vi "ACT_Loop.vi"() -> ()   [LabVIEW 2023, in "Template FX_ACT.lvlib"]
uses:
  Template FX_ACT.lvlib
  RoboRIO Utilities/Global_STOP.vi
  ENUM_ACT_Action.ctl
  ENUM_ACT_State.ctl
  Global_CMD_ACT_Data In.vi
  Global_ACT_Data Out.vi
  Cluster_CMD_ACT_Data.ctl
  <vilib>/Rock Robotics/WPI/MotorControl/WPI_MotorControlType.ctl
  <vilib>/Rock Robotics/SystemInterfaces/DIO/FPGA_DIOPWMChannel.ctl
  <vilib>/Rock Robotics/WPI/PWM/WPI_PWMDeadband.ctl
  <vilib>/Rock Robotics/SystemInterfaces/DIO/FPGA_DIOChannel.ctl
  <vilib>/Rock Robotics/WPI/MotorControl/WPI_MotorControlDeviceRef.ctl
  Shared Code/TypeDefs/Cluser_CAN Data.ctl
  <vilib>/Rock Robotics/WPI/ThirdParty/Phoenix-LabVIEW/Motor Controller/Controls/CTRE_Phoenix_MotorControl_NeutralMode.ctl
  Shared Code/TypeDefs/Cluster_FWD  REV Values.ctl
  Shared Code/TypeDefs/Cluster_Config SRX Motor Output.ctl
  Shared Code/TypeDefs/Cluster_PID Gains.ctl
  Shared Code/TypeDefs/Cluster_SRX SLOT PID Config.ctl
  Shared Code/TypeDefs/Cluster_FX Motion Magic Parameters.ctl
  <vilib>/Rock Robotics/WPI/ThirdParty/Phoenix-LabVIEW/Motor Controller/Controls/CTRE_Phoenix_MotorControl_LimitSwitchNormal.ctl
  Shared Code/TypeDefs/Cluser_Hard Limits.ctl
  Shared Code/TypeDefs/Cluser_Enable-Value I32.ctl
  Shared Code/TypeDefs/Cluser_Config_Soft Limits.ctl
  Shared Code/TypeDefs/Cluser_FX Config_Limit Travel.ctl
  Cluster_Config HW Values.ctl
  b5508d6c-c1cc-4273-80c5-2077d34e1483.vi
  5f725c2a-0ce1-4524-8967-e83b15fdce90.vi
  <vilib>/Rock Robotics/WPI/ThirdParty/Phoenix-LabVIEW/Motor Controller/Controls/CTRE_Phoenix_MotorControl_ControlMode.ctl
  Shared Code/TypeDefs/Cluster_FX CloseLoop Values.ctl
  Shared Code/TypeDefs/Cluster_FX Limit Switchs.ctl
  Shared Code/TypeDefs/Cluster_FX Current Values.ctl
  Cluster_HW Output Values.ctl
  ENUM_CMD_Mode Select.ctl
  Shared Code/TypeDefs/Cluster_FX Sensor Values.ctl
  4f1f8321-3dc8-4b28-8619-20673fc77ec2.vi
  Cluster_SW Output Data.ctl
  Cluster_Config SW Values.ctl
  36677ea0-a1a5-47a3-bc56-4475cb7c281e.vi
  573e44c0-11f4-4bd9-ad56-904ec25dba75.vi
  e7494af9-f670-4352-9dfa-ae6ce50709ea.vi
  6201c2b1-dcd8-4430-86f1-9b4ee56c7753.vi
  Shared Code/TypeDefs/Cluser_FX Config_Current Limits.ctl
  Shared Code/TypeDefs/Cluster_FX_HW All Sensor Values.ctl
  Shared Code/TypeDefs/Cluster_FX Output Set Values.ctl
  Shared Code/TypeDefs/Cluster_High-Low.ctl
panel:
  in  "CMD Override":enum32{"None", "Mode 2", "Mode 1", "STOP"}(tab)
  in  "Mode 2 Data":dbl(slide) scale=-0.2..0.2
  in  "Mode 1 Data":i32
  in  "GO":bool
  out "Current Time":timestamp
  in  "SW Config":T1={"Ver"=0, "Config 1"=0.2}
  out "SW Output":T2
  out "Sensor Read time":dbl format="%.3g"
  out "HW Sensors":T3 {"Set"."Mode" items=["PercentOutput"=0, "Position"=1, "Velocity"=2, "Current"=3, "Follower"=5, "MotionProfile"=6, "MotionMagic"=7, "MotionProfileArc"=10, "Disabled"=15]}
  in  "Read Saved Config":bool
  in  "Update Config":bool
  in  "HW Config":T11 {"TravelLimits"."Soft"."REV"."Counts" format="%#.0f"; "TravelLimits"."Soft"."FWD"."Counts" format="%#.0f"; "Output"."Min"."REV" format="%.2f"; "Output"."Min"."FWD" format="%.2f"; "Output"."Max"."REV" format="%.2f"; "Output"."Max"."FWD" format="%.2f"; "CL"."Max I Accu"."Low" format="%#.8f"; "CL"."Max I Accu"."High" format="%#.8f"; "CL"."Gains"."F" format="%#.8f"; "CL"."Gains"."D" format="%#.8f"; "CL"."Gains"."I" format="%#.8f"; "CL"."Gains"."P" format="%#.8f"; "CL"."Error Allowed"."Low" format="%#.8f"; "CL"."Error Allowed"."High" format="%#.8f"; "CL"."I Zone"."Low" format="%#.8f"; "CL"."I Zone"."High" format="%#.8f"; "CL"."Max Out"."REV" format="%.2f"; "CL"."Max Out"."FWD" format="%.2f"}
  out "CMD":T26
  out "Cycle Time (S)":dbl format="%.3g"
  # "STOP"
  # "Tune Output\nto 1023 Max"
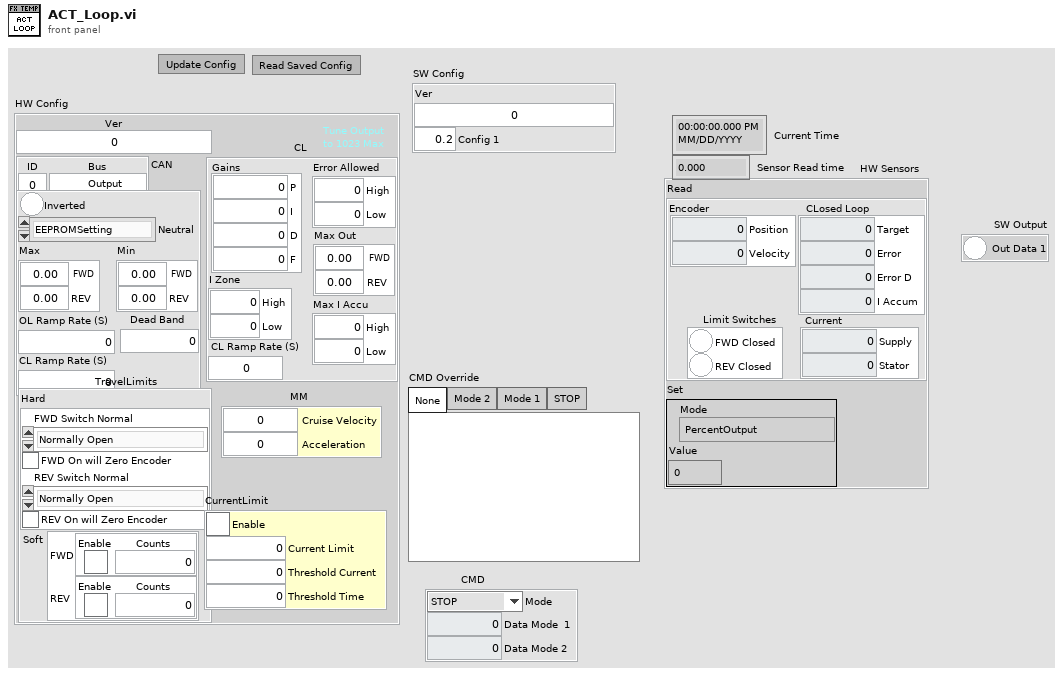
[diagram p1: front panel]
types:
  T1 = typedef "Template FX_ACT.lvlib/Cluster_Config SW Values.ctl" = cluster{"Ver":u64, "Config 1":dbl}
  T2 = typedef "Template FX_ACT.lvlib/Cluster_SW Output Data.ctl" = cluster{"Out Data 1":bool}
  T3 = typedef "Template FX_ACT.lvlib/Cluster_HW Output Values.ctl" = cluster{"Read":T4, "Set":T9}
  T4 = typedef "Cluster_FX_HW All Sensor Values.ctl" = cluster{"Encoder":T5, "CLosed Loop":T6, "Limit Switches":T7, "Current":T8}
  T5 = typedef "Cluster_FX Sensor Values.ctl" = cluster{"Position":i32, "Velocity":i32}
  T6 = typedef "Cluster_FX CloseLoop Values.ctl" = cluster{"Target":dbl, "Error":i32, "Error D":dbl, "I Accum":dbl}
  T7 = typedef "Cluster_FX Limit Switchs.ctl" = cluster{"FWD Closed":bool, "REV Closed":bool}
  T8 = typedef "Cluster_FX Current Values.ctl" = cluster{"Supply":dbl, "Stator":dbl}
  T9 = typedef "Cluster_FX Output Set Values.ctl" = cluster{"Mode":T10, "Value":dbl}
  T10 = typedef "CTRE_Phoenix_MotorControl_ControlMode.ctl" = u16
  T11 = typedef "Template FX_ACT.lvlib/Cluster_Config HW Values.ctl" = cluster{"Ver":u64, "CAN":T12, "Output":T13, "CL":T16, "MM":T19, "TravelLimits":T20, "CurrentLimit":T25}
  T12 = typedef "Cluser_CAN Data.ctl" = cluster{"ID":u8, "Bus":string}
  T13 = typedef "Cluster_Config SRX Motor Output.ctl" = cluster{"Inverted":bool, "Neutral":T14, "Max":T15, "Min":T15, "OL Ramp Rate (S)":dbl, "Dead Band":dbl, "CL Ramp Rate (S)":dbl}
  T14 = typedef "CTRE_Phoenix_MotorControl_NeutralMode.ctl" = enum8{"EEPROMSetting", "Override to Coast", "Override to Brake"}
  T15 = typedef "Cluster_FWD  REV Values.ctl" = cluster{"FWD":dbl, "REV":dbl}
  T16 = typedef "Cluster_PID Config.ctl" = cluster{"Gains":T17, "Error Allowed":T18, "I Zone":T18, "Max Out":T15, "Max I Accu":T18, "CL Ramp Rate (S)":dbl}
  T17 = typedef "Cluster_PID Gains.ctl" = cluster{"P":dbl, "I":dbl, "D":dbl, "F":dbl}
  T18 = typedef "Cluster_High-Low.ctl" = cluster{"High":dbl, "Low":dbl}
  T19 = typedef "Cluster_FX Motion Magic Parameters.ctl" = cluster{"Cruise Velocity":i32, "Acceleration":i32}
  T20 = typedef "Cluser_FX Config_Limit Travel.ctl" = cluster{"Hard":T21, "Soft":T23}
  T21 = typedef "Cluser_Hard Limits.ctl" = cluster{"FWD Switch Normal":T22, "FWD On will Zero Encoder ":bool, "REV Switch Normal":T22, "REV On will Zero Encoder ":bool}
  T22 = typedef "CTRE_Phoenix_MotorControl_LimitSwitchNormal.ctl" = enum16{"Normally Open", "Normally Closed", "Disabled"}
  T23 = typedef "Cluser_Config_Soft Limits.ctl" = cluster{"FWD":T24, "REV":T24}
  T24 = typedef "Cluser_Enable-Value I32.ctl" = cluster{"Enable":bool, "Counts":i32}
  T25 = typedef "Cluser_FX Config_Current Limits.ctl" = cluster{"Enable":bool, "Current Limit":dbl, "Threshold Current":dbl, "Threshold Time":dbl}
  T26 = typedef "Template FX_ACT.lvlib/Cluster_CMD_ACT_Data.ctl" = cluster{"Mode":T27, "Data Mode  1":dbl, "Data Mode 2":dbl}
  T27 = typedef "Template FX_ACT.lvlib/ENUM_CMD_Mode Select.ctl" = enum16{"STOP", "Mode 1", "Mode 2"}
  T28 = typedef "Template FX_ACT.lvlib/Cluster_Config HW Values.ctl" = cluster{"Ver":u64, "CAN":T12, "Output":T29, "CL":T30, "MM":T19, "TravelLimits":T20, "CurrentLimit":T25}
  T29 = typedef "Cluster_Config SRX Motor Output.ctl" = cluster{"Neutral":T14, "Max":T15, "Min":T15, "OL Ramp Rate (S)":dbl, "Dead Band":dbl, "CL Ramp Rate (S)":dbl}
  T30 = typedef "Cluster_SRX SLOT PID Config.ctl" = cluster{"Gains":T17, "Error Allowed":dbl, "I Zone":dbl, "Peak Out 0-1":dbl, "Max I Accu":dbl}
  T31 = typedef "Template FX_ACT.lvlib/ENUM_ACT_State.ctl" = enum16{"Startup", "Configuring", "Stopping", "Moving Mode 1", "Moving Mode 2", "Shutdown"}
  T32 = typedef "WPI_MotorControlDeviceRef.ctl" = cluster{"DeviceStatus":errorcluster, "Type":T33, "PWM":cluster{"PWM Channel":T34, "DeadBand":T35}, "CAN":cluster{"Device Number":u8, "SetOutput VI Ref":variant, "GetOutput VI Ref":variant, "Enable VI Ref":variant, "Disable VI Ref":variant, "Data":variant}, "Invert":bool, "DIO PWM":cluster{"PWM \"Enable\" Channel":T34, "DIOChannel":T36, "PWM Rate":dbl}}
  T33 = typedef "WPI_MotorControlType.ctl" = enum16{"PWM", "CAN", "DIO PWM"}
  T34 = typedef "FPGA_DIOPWMChannel.ctl" = enum8{"PWM 0", "PWM 1", "PWM 2", "PWM 3", "PWM 4", "PWM 5", "PWM 6", "PWM 7", "PWM 8", "PWM 9", "PWM MXP 0", "PWM MXP 1", "PWM MXP 2", "PWM MXP 3", "PWM MXP 4", "PWM MXP 5", "PWM MXP 6", "PWM MXP 7", "PWM MXP 8", "PWM MXP 9", "Invalid"}
  T35 = typedef "WPI_PWMDeadband.ctl" = cluster{"Name":string, "maxPositivePwm":i32, "minPositivePwm":i32, "centerPwm":i32, "maxNegativePwm":i32, "minNegativePwm":i32, "angularRange":u16}
  T36 = typedef "FPGA_DIOChannel.ctl" = enum8{"DIO 0", "DIO 1", "DIO 2", "DIO 3", "DIO 4", "DIO 5", "DIO 6", "DIO 7", "DIO 8", "DIO 9", "DIO MXP 0", "DIO MXP 1", "DIO MXP 2", "DIO MXP 3", "DIO MXP 4", "DIO MXP 5", "DIO MXP 6", "DIO MXP 7", "DIO MXP 8", "DIO MXP 9", "DIO MXP 10", "DIO MXP 11", "DIO MXP 12", "DIO MXP 13", "DIO MXP 14", "DIO MXP 15", "SPI Port CS1", "SPI Port CS2", "SPI Port CS3", "SPI Port MISO", "SPI Port MOSI", "Invalid"}
  T37 = cluster{"Team Files Folder":path, "FX Ref":T32, "State":T31, "Previous State":T31, "Current Time":timestamp, "Previous Time":timestamp, "Start Time":timestamp, "Target Time (ms)":u32, "Cycle Time(S)":dbl, "Update Display":bool, "ACT Input":T26, "HW Config":T28, "SW Config":T1, "Max # Of Config Tries":i32, "HW Out":T3, "SW Out":T2, "CAN Timeout":u32, "FX Mode":T10, "FX Set Value":dbl}
  T38 = typedef "Template FX_ACT.lvlib/ENUM_ACT_Action.ctl" = enum16{"No Action", "Reset Time", "Reset All", "Config HW File Read", "Config HW File Save", "Config SW File Read", "Config SW File Save", "Config From FP", "Config HW Get", "Config HW Set", "Open HW Only", "Control FX Stop", "Control FX Mode 1", "Control FX Mode 2"}
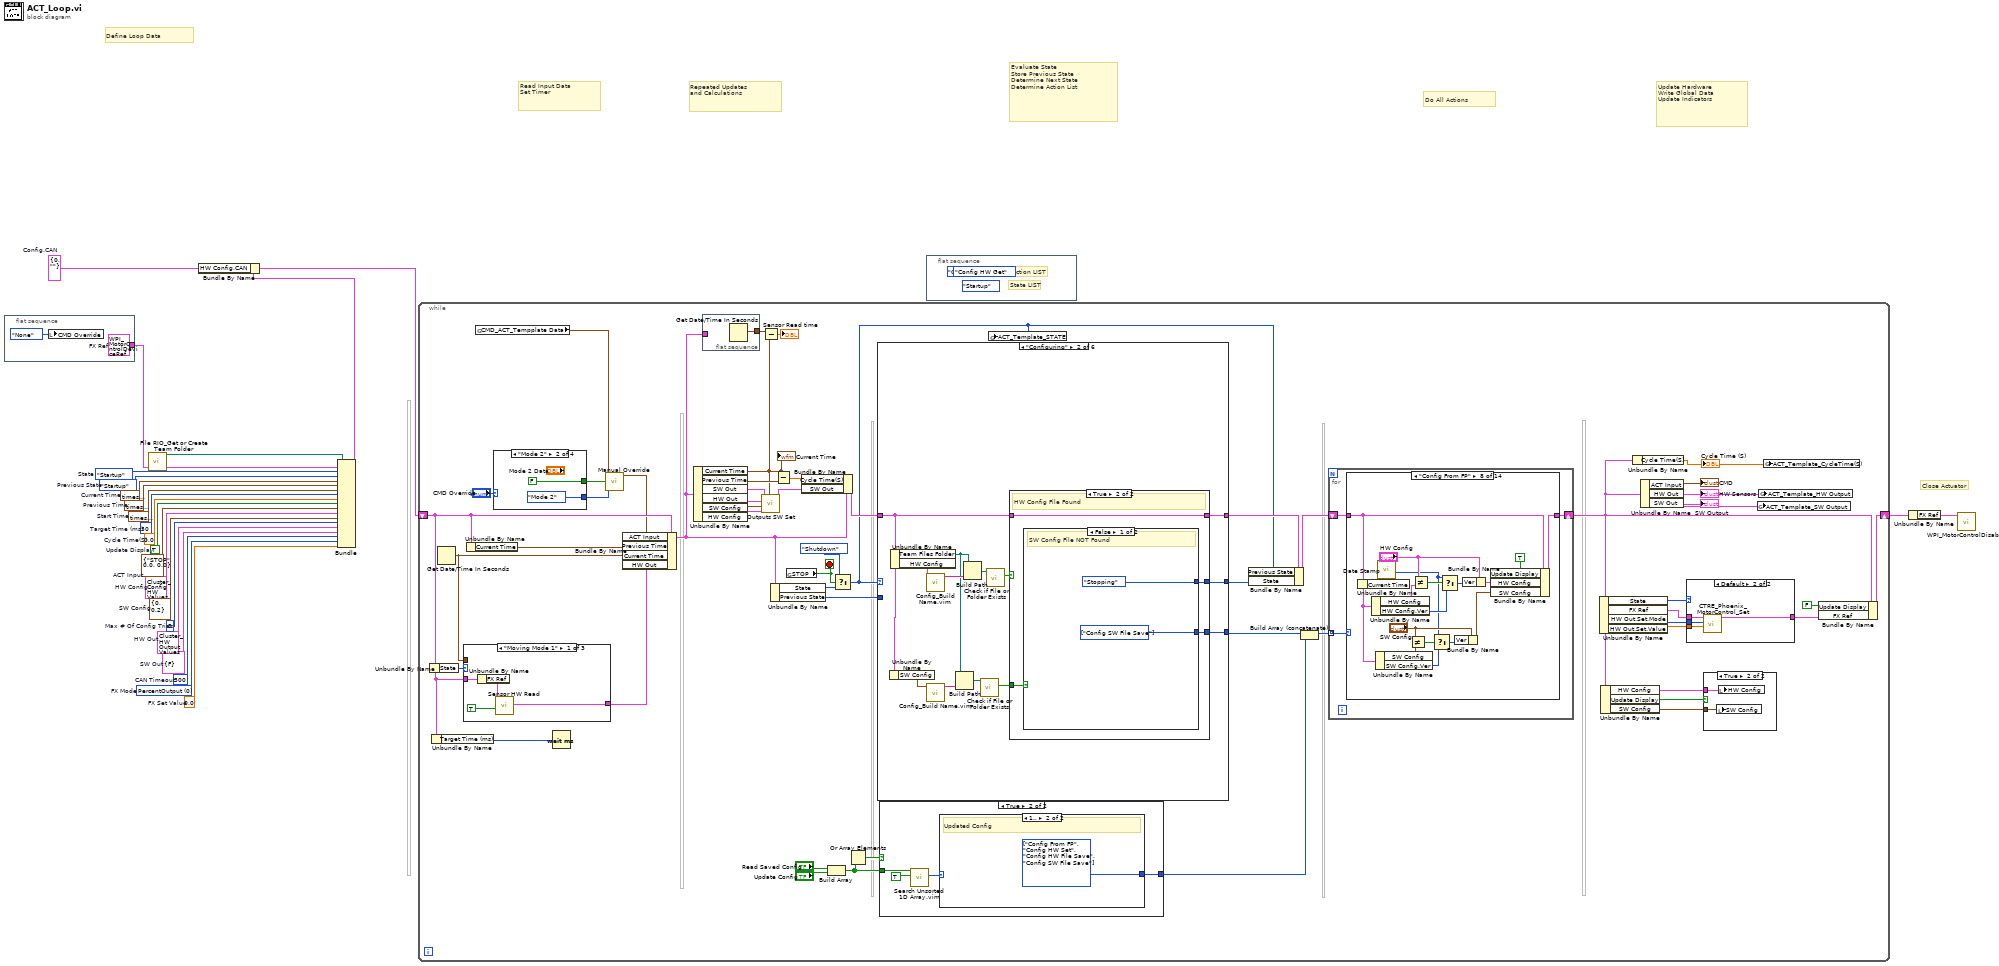
[diagram p0: block diagram]
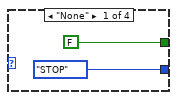
[diagram p2: hidden frame]
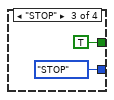
[diagram p3: hidden frame]
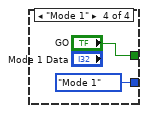
[diagram p4: hidden frame]
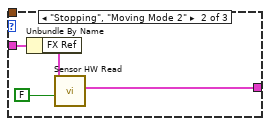
[diagram p5: hidden frame]
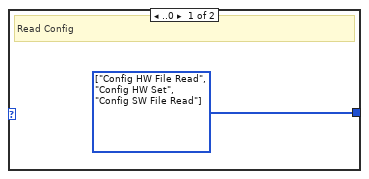
[diagram p8: hidden frame]
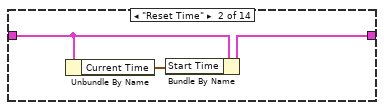
[diagram p10: hidden frame]
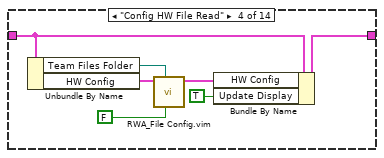
[diagram p12: hidden frame]
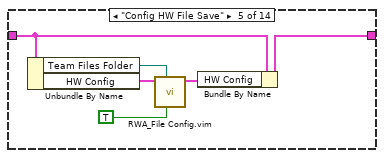
[diagram p13: hidden frame]
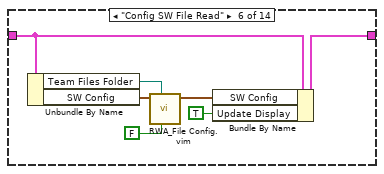
[diagram p14: hidden frame]
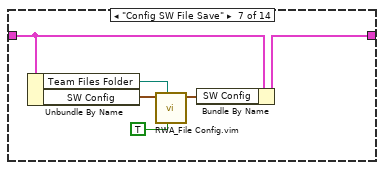
[diagram p15: hidden frame]
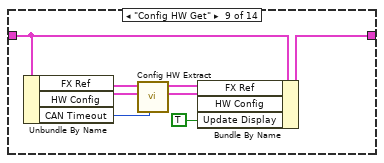
[diagram p16: hidden frame]
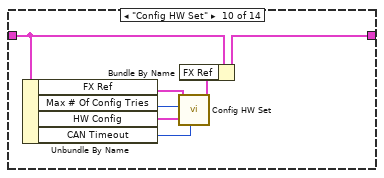
[diagram p17: hidden frame]
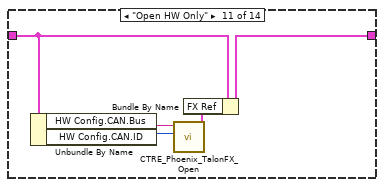
[diagram p18: hidden frame]
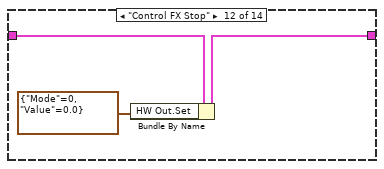
[diagram p19: hidden frame]
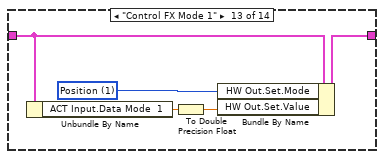
[diagram p20: hidden frame]
diagram:
  w10 = T28 {"Ver"=0, "CAN"={"ID"=0, "Bus"=""}, "Output"={"Neutral"=enum."EEPROMSetting", "Max"={"FWD"=0.0, "REV"=0.0}, "Min"={"FWD"=0.0, "REV"=0.0}, "OL Ramp Rate (S)"=0.0, "Dead Band"=0.0, "CL Ramp Rate (S)"=0.0}, "CL"={"Gains"={"P"=0.0, "I"=0.0, "D"=0.0, "F"=0.0}, "Error Allowed"=0.0, "I Zone"=0.0, "Peak Out 0-1"=0.0, "Max I Accu"=0.0}, "MM"={"Cruise Velocity"=0, "Acceleration"=0}, "TravelLimits"={"Hard"={"FWD Switch Normal"=enum."Normally Open", "FWD On will Zero Encoder "=FALSE, "REV Switch Normal"=enum."Normally Open", "REV On will Zero Encoder "=FALSE}, "Soft"={"FWD"={"Enable"=FALSE, "Counts"=0}, "REV"={"Enable"=FALSE, "Counts"=0}}}, "CurrentLimit"={"Enable"=FALSE, "Current Limit"=0.0, "Threshold Current"=0.0, "Threshold Time"=0.0}}  # HW Config
  w7 = T2 {"Out Data 1"=FALSE}  # SW Out
  w9 = T1 {"Ver"=0, "Config 1"=0.2}  # SW Config
  w8 = T3 {"Read"={"Encoder"={"Position"=0, "Velocity"=0}, "CLosed Loop"={"Target"=0.0, "Error"=0, "Error D"=0.0, "I Accum"=0.0}, "Limit Switches"={"FWD Closed"=FALSE, "REV Closed"=FALSE}, "Current"={"Supply"=0.0, "Stator"=0.0}}, "Set"={"Mode"=0, "Value"=0.0}}  # HW Out
  w3 = 0.0  # FX Set Value
  w4 = T10 0 items=["PercentOutput"=0, "Position"=1, "Velocity"=2, "Current"=3, "Follower"=5, "MotionProfile"=6, "MotionMagic"=7, "MotionProfileArc"=10, "Disabled"=15]  # FX Mode
  w2 = u32 300  # CAN Timeout
  w1 = 3  # Max # Of Config Tries
  w12 = TRUE  # Update Display
  w13 = T12 {"ID"=0, "Bus"=""}  # Config.CAN
  w18 = 0.0  # Cycle Time(S)
  w19 = ENUM_ACT_State."Startup"  # Previous State
  w20 = timestamp(0 s since 1904-01-01)  # Previous Time
  w21 = u32 50  # Target Time (ms)
  w6 = T26 {"Mode"=enum."STOP", "Data Mode  1"=0.0, "Data Mode 2"=0.0}  # ACT Input
  w22 = timestamp(0 s since 1904-01-01)  # Start Time
  w23 = timestamp(0 s since 1904-01-01)  # Current Time
  w24 = ENUM_ACT_State."Startup"  # State
  # "Close Actuator"
  # "Define Loop Data"
  # "Repeated Updates\nand Calculations"
  # "Read Input Data\nSet Timer"
  # "Evaluate State\nStore Previous State\nDetermine Next State\nDetermine Action List"
  # "Do All Actions"
  # "Update Hardware\nWrite Global Data\nUpdate Indicators"
  n1 = flat-sequence {
    tunnel: [w26] -> w14
    frame #0 {
      w26 = T32 {"DeviceStatus"={"status"=FALSE, "code"=0, "source"=""}, "Type"=enum."PWM", "PWM"={"PWM Channel"=enum."PWM 1", "DeadBand"={"Name"="", "maxPositivePwm"=0, "minPositivePwm"=0, "centerPwm"=0, "maxNegativePwm"=0, "minNegativePwm"=0, "angularRange"=0}}, "CAN"={"Device Number"=0, "SetOutput VI Ref"=variant(enum8{"Percent VBus", "Current", "Speed", "Position", "Voltage"} enum."Percent VBus"), "GetOutput VI Ref"=variant(refnum<k1> refnum), "Enable VI Ref"=variant(dbl 12.0), "Disable VI Ref"=variant(enum8{"Percent VBus", "Speed", "Position", "Slave", "Unchanged / Invalid", "Voltage Compensation", "Current", "Motion Profile"} enum."Percent VBus"), "Data"=variant}, "Invert"=FALSE, "DIO PWM"={"PWM \"Enable\" Channel"=enum."Invalid", "DIOChannel"=enum."Invalid", "PWM Rate"=0.0}}  # FX Ref
      n2 = local write "CMD Override"(enum32{"None", "Mode 2", "Mode 1", "STOP"}."None" ("CMD Override")) -> ()
    }
  }
  n3 = call "File RIO_Get or Create Team Folder.vi"() -> ("Team Files Folder"=w5:path)  [unwired: 10 in, 1 out]
  n4 = Bundle("Team Files Folder"=w5, "FX Ref"=w14, "State"=w24, "Previous State"=w19, "Current Time"=w23, "Previous Time"=w20, "Start Time"=w22, "Target Time (ms)"=w21, "Cycle Time(S)"=w18, "Update Display"=w12, "ACT Input"=w6, "HW Config"=w10, "SW Config"=w9, "Max # Of Config Tries"=w1, "HW Out"=w8, "SW Out"=w7, "CAN Timeout"=w2, "FX Mode"=w4, "FX Set Value"=w3) -> (w16:T37)  [unwired: 1 in]
  n5 = Bundle By Name(cluster=w16, "HW Config.CAN"=w13) -> (w15:T37)
  n6 = while {
    shift-right: [w63] -> w17
    shift-left: w15 -> [w33]
    stop <- w76 stop-if-true
    n7 = Unbundle By Name(w33) -> ("State"=w53:T31)
    n8 = Unbundle By Name(w33) -> ("Target Time (ms)"=w73:u32)
    n9 = Get Date/Time In Seconds() -> (seconds since 1Jan1904=w49:timestamp)
    n10 = case shown="\"Moving Mode 1\"" w53 {
      tunnel: w33 -> [w92 w96 _]
      tunnel: w49 -> [_ _ _]
      tunnel: [w89 w93 _] -> w34
      frame "Moving Mode 1" {
        n11 = Unbundle By Name(w92) -> ("FX Ref"=w91:T32)
        n12 = call "Sensor HW Read.vi"("Read Closed Loop"=TRUE, "Ref"=w91) -> ("Sensor Values Out"=w89:T3)  [unwired: 7 in, 2 out]
      }
      frame "Stopping", "Moving Mode 2" {
        n13 = Unbundle By Name(w96) -> ("FX Ref"=w95:T32)
        n14 = call "Sensor HW Read.vi"("Read Closed Loop"=FALSE, "Ref"=w95) -> ("Sensor Values Out"=w93:T3)  [unwired: 7 in, 2 out]
      }
      frame "Startup", "Configuring", "Shutdown" {
      }
    }
    n15 = Unbundle By Name(w33) -> ("Current Time"=w72:timestamp)
    n16 = global read "Global_CMD_ACT_Data In.vi" "CMD_ACT_Tempplate Data"() -> (w31:T26)
    n17 = case shown="\"Mode 2\"" "CMD Override" {
      tunnel: [FALSE ("Enable") FALSE ("Enable") TRUE ("Positon GO") "GO"] -> w29
      tunnel: [ENUM_CMD_Mode_Select."STOP" ("Override") ENUM_CMD_Mode_Select."Mode 2" ("Override") ENUM_CMD_Mode_Select."STOP" ("Override") ENUM_CMD_Mode_Select."Mode 1" ("Override")] -> w28
      frame "None" {
      }
      frame "Mode 2" {
      }
      frame "STOP" {
      }
      frame "Mode 1" {
      }
    }
    n18 = Wait (ms)(milliseconds to wait=w73) -> ()  [unwired: 1 out]
    n19 = call "Manual Override.vi"("Override"=w28, "Enable"=w29, "Auto CMD"=w31) -> ("OverRide Command Out"=w32:T26)  [unwired: 8 in]
    n20 = Bundle By Name(cluster=w33, "ACT Input"=w32, "Previous Time"=w72, "Current Time"=w49, "HW Out"=w34) -> (w35:T37)
    n21 = Unbundle By Name(w35) -> ("Current Time"=w39:timestamp, "Previous Time"=w70:timestamp, "SW Out"=w42:T2, "HW Out"=w40:T3, "SW Config"=w38:T1, "HW Config"=w37:T28)
    "Current Time" <- w39
    n22 = flat-sequence {
      tunnel: [w88] -> w51
      tunnel: w35 -> [_]
      frame #0 {
        n23 = Get Date/Time In Seconds() -> (seconds since 1Jan1904=w88:timestamp)
      }
    }
    n24 = call "Outputs SW Set.vi"("Current Time"=w39, "HW Config"=w37, "SW Config"=w38, "Sensor Values"=w40, "SW Output"=w42) -> ("SW Output Out"=w41:T2)  [unwired: 6 in]
    n25 = Subtract(x=w51, y=w39) -> (x-y=→"Sensor Read time":dbl)
    n26 = Unbundle By Name(w35) -> ("State"=w74:T31, "Previous State"=w71:T31)
    n27 = Subtract(x=w39, y=w70) -> (x-y=w68:dbl)
    n28 = global read "Global_STOP.vi" "STOP"() -> (w76:bool)
    n29 = Bundle By Name(cluster=w35, "Cycle Time(S)"=w68, "SW Out"=w41) -> (w69:T37)
    n30 = Build Array("Read Saved Config", "Update Config") -> (w45:bool[])
    n31 = Select(t=ENUM_ACT_State."Shutdown" ("State"), s=w76, f=w74) -> (s? t:f=w27:T31)
    n32 = Or Array Elements(Boolean array=w45) -> (logical OR=w46:bool)
    n33 = case shown="\"Configuring\"" w27 {
      selector: w27 -> [_ _ _ w230 w246 _]
      tunnel: w69 -> [w188 w194 w217 w231 w247 w262]
      tunnel: [w188 w197 w216 w232 w248 w262] -> w78
      tunnel: [ENUM_ACT_State."Configuring" ("State") w196 w215 w234 w250 ENUM_ACT_State."Shutdown" ("State")] -> w77
      tunnel: [w187 w195 w213 w229 w244 w260] -> w67
      tunnel: w71 -> [_ _ _ _ _ _]
      frame "Startup" {
        w187 = T38[] [enum."Reset Time"] items=["No Action", "Reset Time", "Reset All", "Config HW File Read", "Config HW File Save", "Config SW File Read", "Config SW File Save", "Config From FP", "Config HW Get", "Config HW Set", "Open HW Only", "Control FX Stop", "Control FX Mode 1", "Control FX Mode 2"] ("Actions")
      }
      frame "Configuring" {
        n34 = Unbundle By Name(w194) -> ("SW Config"=w192:T1)
        n35 = Unbundle By Name(w194) -> ("Team Files Folder"=w191:path, "HW Config"=w199:T28)
        n36 = call "Config_Build Name.vim"("Config First Name"=w199) -> ("Cfg file"=w201:string)  [unwired: 9 in, 1 out]
        n37 = call "Config_Build Name.vim"("Config First Name"=w192) -> ("Cfg file"=w193:string)  [unwired: 9 in, 1 out]
        n38 = Build Path(base path=w191, name or relative path=w193) -> (appended path=w190:path)
        n39 = Build Path(base path=w191, name or relative path=w201) -> (appended path=w200:path)
        n40 = call <vilib>:"Check if File or Folder Exists.vi"("path"=w190) -> ("file or folder exists?"=w189:bool)  [unwired: 8 in, 2 out]
        n41 = call <vilib>:"Check if File or Folder Exists.vi"("path"=w200) -> ("file or folder exists?"=w198:bool)  [unwired: 8 in, 2 out]
        n42 = case shown="True" w198 {
          tunnel: w194 -> [w204 w208]
          tunnel: [w204 w208] -> w197
          tunnel: [ENUM_ACT_State."Configuring" ("State") w207] -> w196
          tunnel: [w202 w206] -> w195
          tunnel: w189 -> [_ w205]
          frame False {
            w202 = T38[] [enum."Open HW Only", enum."Config HW Get", enum."Config HW File Save"] items=["No Action", "Reset Time", "Reset All", "Config HW File Read", "Config HW File Save", "Config SW File Read", "Config SW File Save", "Config From FP", "Config HW Get", "Config HW Set", "Open HW Only", "Control FX Stop", "Control FX Mode 1", "Control FX Mode 2"] ("Actions")
            # "HW Config File Not Found"
          }
          frame True {
            # "HW Config File Found"
            n43 = case shown="False" w205 {
              tunnel: [ENUM_ACT_State."Stopping" ("State") ENUM_ACT_State."Stopping" ("State")] -> w207
              tunnel: [w209 w211] -> w206
              frame False {
                w209 = T38[] [enum."Config SW File Save"] items=["No Action", "Reset Time", "Reset All", "Config HW File Read", "Config HW File Save", "Config SW File Read", "Config SW File Save", "Config From FP", "Config HW Get", "Config HW Set", "Open HW Only", "Control FX Stop", "Control FX Mode 1", "Control FX Mode 2"] ("Actions")
                # "SW Config File NOT Found"
              }
              frame True {
                w211 = T38[] [enum."Config HW File Read", enum."Config HW Set", enum."Config SW File Read", enum."Reset All", enum."Control FX Stop"] items=["No Action", "Reset Time", "Reset All", "Config HW File Read", "Config HW File Save", "Config SW File Read", "Config SW File Save", "Config From FP", "Config HW Get", "Config HW Set", "Open HW Only", "Control FX Stop", "Control FX Mode 1", "Control FX Mode 2"] ("Actions")
                # "SW Config File Found"
              }
            }
          }
        }
      }
      frame "Stopping" {
        (unwired) TRUE
        w214 = T38[] [enum."Control FX Stop"] items=["No Action", "Reset Time", "Reset All", "Config HW File Read", "Config HW File Save", "Config SW File Read", "Config SW File Save", "Config From FP", "Config HW Get", "Config HW Set", "Open HW Only", "Control FX Stop", "Control FX Mode 1", "Control FX Mode 2"] ("Actions")
        n44 = Unbundle By Name(w217) -> ("ACT Input.Mode"=w218:T27)
        n45 = case shown="\"STOP\"" w218 {
          tunnel: w217 -> [w221 w224 w227]
          tunnel: [w221 w224 w227] -> w216
          tunnel: [ENUM_ACT_State."Stopping" ("State") ENUM_ACT_State."Moving Mode 1" ("State") ENUM_ACT_State."Moving Mode 2" ("State")] -> w215
          tunnel: [w219 w222 w225] -> w213
          tunnel: w214 -> [w219 w222 w225]
          frame "STOP" {
          }
          frame "Mode 1" {
          }
          frame "Mode 2" {
          }
        }
      }
      frame "Moving Mode 1" {
        w228 = T38[] [enum."Control FX Stop"] items=["No Action", "Reset Time", "Reset All", "Config HW File Read", "Config HW File Save", "Config SW File Read", "Config SW File Save", "Config From FP", "Config HW Get", "Config HW Set", "Open HW Only", "Control FX Stop", "Control FX Mode 1", "Control FX Mode 2"] ("Actions")
        n46 = Unbundle By Name(w231) -> ("ACT Input.Mode"=w233:T27)
        n47 = case shown="\"Mode 2\"" w233 {
          tunnel: [ENUM_ACT_State."Stopping" ("State") ENUM_ACT_State."Moving Mode 2" ("State") w242] -> w234
          tunnel: w231 -> [w237 w240 w243]
          tunnel: [w237 w240 w243] -> w232
          tunnel: w230 -> [_ _ w242]
          tunnel: [w235 w238 w241] -> w229
          tunnel: w228 -> [w235 w238 _]
          frame "STOP" {
          }
          frame "Mode 2" {
          }
          frame "Mode 1" {
            w241 = T38[] [enum."Control FX Mode 1"] items=["No Action", "Reset Time", "Reset All", "Config HW File Read", "Config HW File Save", "Config SW File Read", "Config SW File Save", "Config From FP", "Config HW Get", "Config HW Set", "Open HW Only", "Control FX Stop", "Control FX Mode 1", "Control FX Mode 2"] ("Actions")
          }
        }
      }
      frame "Moving Mode 2" {
        w245 = T38[] [enum."Control FX Stop"] items=["No Action", "Reset Time", "Reset All", "Config HW File Read", "Config HW File Save", "Config SW File Read", "Config SW File Save", "Config From FP", "Config HW Get", "Config HW Set", "Open HW Only", "Control FX Stop", "Control FX Mode 1", "Control FX Mode 2"] ("Actions")
        n48 = Unbundle By Name(w247) -> ("ACT Input.Mode"=w249:T27)
        n49 = case shown="\"Mode 2\"" w249 {
          tunnel: [ENUM_ACT_State."Stopping" ("State") w254 ENUM_ACT_State."Moving Mode 1" ("State")] -> w250
          tunnel: w247 -> [w253 w256 w259]
          tunnel: [w253 w256 w259] -> w248
          tunnel: w246 -> [_ w254 _]
          tunnel: [w251 w255 w257] -> w244
          tunnel: w245 -> [w251 _ w257]
          frame "STOP" {
          }
          frame "Mode 2" {
            w255 = T38[] [enum."Control FX Mode 2"] items=["No Action", "Reset Time", "Reset All", "Config HW File Read", "Config HW File Save", "Config SW File Read", "Config SW File Save", "Config From FP", "Config HW Get", "Config HW Set", "Open HW Only", "Control FX Stop", "Control FX Mode 1", "Control FX Mode 2"] ("Actions")
          }
          frame "Mode 1" {
          }
        }
      }
      frame "Shutdown" {
        w260 = T38[] [enum."Reset All"] items=["No Action", "Reset Time", "Reset All", "Config HW File Read", "Config HW File Save", "Config SW File Read", "Config SW File Save", "Config From FP", "Config HW Get", "Config HW Set", "Open HW Only", "Control FX Stop", "Control FX Mode 1", "Control FX Mode 2"] ("Actions")
      }
    }
    n50 = case shown="True" w46 {
      tunnel: w45 -> [_ w99]
      tunnel: [_ w97] -> w44
      frame False {
      }
      frame True {
        n51 = call "Search Unsorted 1D Array.vim"("element"=TRUE, "unsorted 1D array"=w99) -> ("index of element"=w98:i32)  [unwired: 9 in]
        n52 = case shown="1.." w98 {
          tunnel: [w101 w102] -> w97
          frame ..0 {
            w101 = T38[] [enum."Config HW File Read", enum."Config HW Set", enum."Config SW File Read"] items=["No Action", "Reset Time", "Reset All", "Config HW File Read", "Config HW File Save", "Config SW File Read", "Config SW File Save", "Config From FP", "Config HW Get", "Config HW Set", "Open HW Only", "Control FX Stop", "Control FX Mode 1", "Control FX Mode 2"] ("Actions")
            # "Read Config"
          }
          frame 1.. {
            w102 = T38[] [enum."Config From FP", enum."Config HW Set", enum."Config HW File Save", enum."Config SW File Save"] items=["No Action", "Reset Time", "Reset All", "Config HW File Read", "Config HW File Save", "Config SW File Read", "Config SW File Save", "Config From FP", "Config HW Get", "Config HW Set", "Open HW Only", "Control FX Stop", "Control FX Mode 1", "Control FX Mode 2"] ("Actions")
            # "Updated Config"
          }
        }
      }
    }
    n53 = global write "Global_ACT_Data Out.vi" "ACT_Template_STATE"(w27) -> ()
    n54 = Bundle By Name(cluster=w78, "Previous State"=w27, "State"=w77) -> (w79:T37)
    n55 = Build Array (concatenate)(w67, w44) -> (w61:T38[])
    n56 = for {
      tunnel: w61 -> [w105] mode=indexing
      shift-right: [w104] -> w60
      shift-left: w79 -> [w103]
      n57 = case shown="\"Config From FP\"" w105 {
        tunnel: w103 -> [w106 w109 w110 w116 w122 w129 w135 w143 w158 w166 w170 w175 w179 w183]
        tunnel: [w106 w108 w110 w117 w123 w130 w136 w153 w159 w167 w171 w176 w181 w185] -> w104
        frame "No Action" {
        }
        frame "Reset Time" {
          n58 = Unbundle By Name(w109) -> ("Current Time"=w107:timestamp)
          n59 = Bundle By Name(cluster=w109, "Start Time"=w107) -> (w108:T37)
        }
        frame "Reset All" {
        }
        frame "Config HW File Read" {
          n60 = Unbundle By Name(w116) -> ("Team Files Folder"=w113:path, "HW Config"=w115:T28)
          n61 = call "RWA_File Config.vim"("Read(f) Save(t)"=FALSE ("Read(f) Write(t)"), "Target Folder Folder"=w113, "Any Config"=w115) -> ("Any Config Out"=w114:T28)  [unwired: 4 in, 4 out]
          n62 = Bundle By Name(cluster=w116, "HW Config"=w114, "Update Display"=TRUE) -> (w117:T37)
        }
        frame "Config HW File Save" {
          n63 = Unbundle By Name(w122) -> ("Team Files Folder"=w119:path, "HW Config"=w121:T28)
          n64 = call "RWA_File Config.vim"("Read(f) Save(t)"=TRUE ("Read(f) Write(t)"), "Target Folder Folder"=w119, "Any Config"=w121) -> ("Any Config Out"=w120:T28)  [unwired: 4 in, 4 out]
          n65 = Bundle By Name(cluster=w122, "HW Config"=w120) -> (w123:T37)
        }
        frame "Config SW File Read" {
          n66 = Unbundle By Name(w129) -> ("Team Files Folder"=w126:path, "SW Config"=w128:T1)
          n67 = call "RWA_File Config.vim"("Read(f) Save(t)"=FALSE ("Read(f) Write(t)"), "Target Folder Folder"=w126, "Any Config"=w128) -> ("Any Config Out"=w127:T1)  [unwired: 4 in, 4 out]
          n68 = Bundle By Name(cluster=w129, "SW Config"=w127, "Update Display"=TRUE) -> (w130:T37)
        }
        frame "Config SW File Save" {
          n69 = Unbundle By Name(w135) -> ("Team Files Folder"=w132:path, "SW Config"=w134:T1)
          n70 = call "RWA_File Config.vim"("Read(f) Save(t)"=TRUE ("Read(f) Write(t)"), "Target Folder Folder"=w132, "Any Config"=w134) -> ("Any Config Out"=w133:T1)  [unwired: 4 in, 4 out]
          n71 = Bundle By Name(cluster=w135, "SW Config"=w133) -> (w136:T37)
        }
        frame "Config From FP" {
          n72 = Unbundle By Name(w143) -> ("Current Time"=w152:timestamp)
          n73 = Unbundle By Name(w143) -> ("HW Config"=w142:T28, "HW Config.Ver"=w139:u64)
          n74 = Unbundle By Name(w143) -> ("SW Config"=w145:T1, "SW Config.Ver"=w147:u64)
          n75 = call "Date Stamp.vi"("Time"=w152) -> ("U64 Out"=w138:u64)  [unwired: 5 in, 1 out]
          n76 = Not Equal?(x=w145, y="SW Config") -> (x != y?=w148:bool)
          n77 = Not Equal?(x="HW Config", y=w142) -> (x != y?=w140:bool)
          n78 = Select(t=w138, s=w148, f=w147) -> (s? t:f=w146:u64)
          n79 = Select(t=w138, s=w140, f=w139) -> (s? t:f=w137:u64)
          n80 = Bundle By Name(cluster="SW Config", "Ver"=w146) -> (w150:T1)
          n81 = Bundle By Name(cluster="HW Config", "Ver"=w137) -> (w151:T11)
          n82 = Bundle By Name(cluster=w143, "Update Display"=TRUE, "HW Config"=w151, "SW Config"=w150) -> (w153:T37)
        }
        frame "Config HW Get" {
          n83 = Unbundle By Name(w158) -> ("FX Ref"=w161:T32, "HW Config"=w160:T28, "CAN Timeout"=w154:u32)
          n84 = call "Config HW Extract.vi"("Send Cmd Timout(ms)"=w154, "Wrist Config"=w160, "DevRef"=w161) -> ("Wrist Config Data Out"=w156:T11, "DevRef Out"=w157:T32)  [unwired: 6 in, 1 out]
          n85 = Bundle By Name(cluster=w158, "FX Ref"=w157, "HW Config"=w156, "Update Display"=TRUE) -> (w159:T37)
        }
        frame "Config HW Set" {
          n86 = Unbundle By Name(w166) -> ("FX Ref"=w168:T32, "Max # Of Config Tries"=w162:i32, "HW Config"=w164:T28, "CAN Timeout"=w163:u32)
          n87 = call "Config HW Set.vi"("Send Cmd Timout(ms)"=w163, "Wrist Config"=w164, "Max # Of Tries"=w162, "DevRef"=w168) -> ("DevRef Out Out"=w165:T32)  [unwired: 6 in, 1 out]
          n88 = Bundle By Name(cluster=w166, "FX Ref"=w165) -> (w167:T37)
        }
        frame "Open HW Only" {
          n89 = Unbundle By Name(w170) -> ("HW Config.CAN.Bus"=w169:string, "HW Config.CAN.ID"=w173:u8)
          n90 = call <vilib>:"CTRE_Phoenix_TalonFX_Open.vi"("Device Number"=w173, "CAN Bus"=w169) -> ("PhoenixMotorControlDevRef"=w172:T32)  [unwired: 8 in, 1 out]
          n91 = Bundle By Name(cluster=w170, "FX Ref"=w172) -> (w171:T37)
        }
        frame "Control FX Stop" {
          n92 = Bundle By Name(cluster=w175, "HW Out.Set"=T9 {"Mode"=0, "Value"=0.0}) -> (w176:T37)
        }
        frame "Control FX Mode 1" {
          w180 = T10 1 items=["PercentOutput"=0, "Position"=1, "Velocity"=2, "Current"=3, "Follower"=5, "MotionProfile"=6, "MotionMagic"=7, "MotionProfileArc"=10, "Disabled"=15] ("FX Mode")
          n93 = Unbundle By Name(w179) -> ("ACT Input.Data Mode  1"=w177:dbl)
          n94 = To Double Precision Float(number=w177) -> (double precision float=w178:dbl)
          n95 = Bundle By Name(cluster=w179, "HW Out.Set.Mode"=w180, "HW Out.Set.Value"=w178) -> (w181:T37)
        }
        frame "Control FX Mode 2" {
          w184 = T10 0 items=["PercentOutput"=0, "Position"=1, "Velocity"=2, "Current"=3, "Follower"=5, "MotionProfile"=6, "MotionMagic"=7, "MotionProfileArc"=10, "Disabled"=15] ("FX Mode")
          n96 = Unbundle By Name(w183) -> ("ACT Input.Data Mode 2"=w182:dbl)
          n97 = Bundle By Name(cluster=w183, "HW Out.Set.Mode"=w184, "HW Out.Set.Value"=w182) -> (w185:T37)
        }
      }
    }
    n98 = Unbundle By Name(w60) -> ("State"=w54:T31, "FX Ref"=w65:T32, "HW Out.Set.Mode"=w55:T10, "HW Out.Set.Value"=w56:dbl)
    n99 = Unbundle By Name(w60) -> ("HW Config"=w57:T28, "Update Display"=w58:bool, "SW Config"=w36:T1)
    n100 = Unbundle By Name(w60) -> ("Cycle Time(S)"=w62:dbl)
    "Cycle Time (S)" <- w62
    n101 = Unbundle By Name(w60) -> ("ACT Input"=→"CMD":T26, "HW Out"=w52:T3, "SW Out"=w43:T2)
    "HW Sensors" <- w52
    "SW Output" <- w43
    n102 = case shown="Default" w54 {
      tunnel: w65 -> [w263 w267]
      tunnel: [w263 w266] -> w64
      tunnel: w56 -> [_ w265]
      tunnel: w55 -> [_ w264]
      frame "Startup", "Configuring" {
      }
      frame Default {
        n103 = call <vilib>:"CTRE_Phoenix_MotorControl_Set.vi"("Output"=w265, "Control Mode"=w264, "PhoenixMotorControlDevRef"=w267) -> ("PhoenixMotorControlDevRef"=w266:T32)  [unwired: 7 in, 1 out]
      }
    }
    n104 = case shown="True" w58 {
      tunnel: w57 -> [_ w269]
      tunnel: w36 -> [_ w268]
      frame False {
      }
      frame True {
        n105 = local write "SW Config"(w268) -> ()
        n106 = local write "HW Config"(w269) -> ()
      }
    }
    n107 = global write "Global_ACT_Data Out.vi" "ACT_Template_SW Output"(w43) -> ()
    n108 = global write "Global_ACT_Data Out.vi" "ACT_Template_HW Output"(w52) -> ()
    n109 = global write "Global_ACT_Data Out.vi" "ACT_Template_CycleTime(S)"(w62) -> ()
    n110 = Bundle By Name(cluster=w60, "Update Display"=FALSE, "FX Ref"=w64) -> (w63:T37)
  }
  n111 = flat-sequence {
    frame #0 {
      (unwired) ENUM_ACT_Action."Open HW Only" ("Action")
      (unwired) ENUM_ACT_State."Startup" ("State")
      (unwired) ENUM_ACT_Action."Config HW Get" ("Action")
      # "State LIST"
      # "Action LIST"
    }
  }
  n112 = Unbundle By Name(w17) -> ("FX Ref"=w11:T32)
  n113 = call <vilib>:"WPI_MotorControlDisable.vi"("MotorControlDevRef"=w11) -> ()  [unwired: 9 in, 2 out]
